vi "Conclude.vi"(8 "error in (no error)":errorcluster, 10 "Iterator Settings":T1={"Prepare timeout (ms)"=200, "Iterate timeout (ms)"=50, "Conclude timeout (ms)"=200, "Iterate period (ms)"=200, "Number of iterations"=5, "Time before stop (ms)"=5, "Active Stop Conditions"={"Number of Iterations"=FALSE, "Time Elapsed"=FALSE, "Iteration Result"=FALSE}, "Prepare Msg"=refnum, "Iterate Msg"=refnum, "Conclude Msg"=refnum, "Iterations End Report"=refnum}, 11 "Iterator Actor in":refnum<class "Iterator Actor.lvclass">) -> (0 "error out":errorcluster, 3 "Iterator Actor out":refnum<class "Iterator Actor.lvclass">)   [LabVIEW 2023, in "Iterator Actor.lvlib" / "Iterator Actor.lvclass"]
doc: "Calls the Conclude method of the Client."
uses:
  Iterator Actor.lvclass
  Abstract Iterator Actor/Iterator Settings.ctl
  Iterator Actor Abstract Messages/Iterator Report Iterations End Msg/Iterator Report Iterations End Msg.lvclass
  <vilib>/ActorFramework/Message/Message.lvclass
  Abstract Iterator Actor/Active Stop Conditions.ctl
  <vilib>/ActorFramework/Actor/Actor.lvclass/Actor.ctl
  Iterator Actor Abstract Messages/Iterator Reply Msg/Iterator Reply Msg.lvclass
  Iterator Actor Abstract Messages/Iterator Reply Msg/Iterator Reply Msg.lvclass/Iterator Reply Msg.ctl
  <vilib>/ActorFramework/Message Enqueuer/Message Enqueuer.lvclass/Message Enqueuer.ctl
  <vilib>/ActorFramework/Message Enqueuer/Enqueue.vi
  <vilib>/ActorFramework/Message Priority Queue/Priority Enqueue.vi
  Iterator Actor.lvclass/Iterator Actor.ctl
  <vilib>/ActorFramework/Actor/Actor.lvclass
  <vilib>/ErrorRing/Error Ring.xnode
  C:/Projects/Iterator Actor/Abstract Iterator Actor/Abstract Iterator Actor.lvclass
  C:/Program Files/National Instruments/LabVIEW 2023/vi.lib/LS Instruments AG/Async Methods Actor/Async Methods Actor/Async Methods Actor/Async Methods Actor.lvclass
  C:/Program Files/National Instruments/LabVIEW 2023/vi.lib/ActorFramework/Actor/Actor.lvclass
  C:/Projects/Iterator Actor/Iterator Actor/Iterator Actor/Iterator Actor.lvclass
  <vilib>/Utility/error.llb/Error Cluster From Error Code.vi
  Abstract Iterator Actor/Abstract Iterator Actor.lvclass
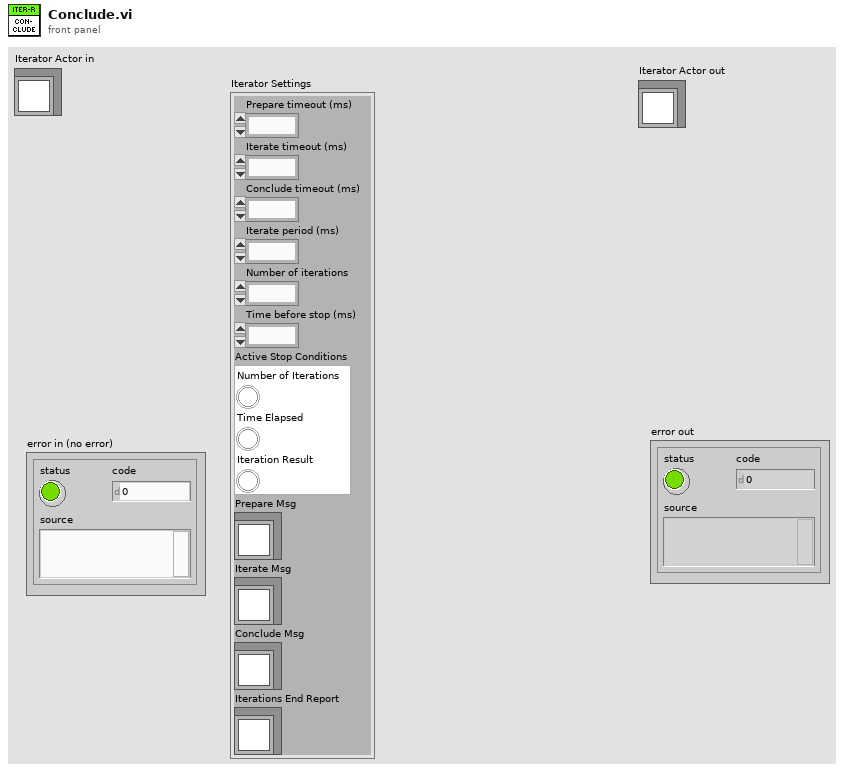
[diagram p1: front panel]
types:
  T1 = typedef "Iterator Actor.lvlib/Abstract Iterator Actor.lvclass/Iterator Settings.ctl" = cluster{"Prepare timeout (ms)":i32, "Iterate timeout (ms)":i32, "Conclude timeout (ms)":i32, "Iterate period (ms)":i32, "Number of iterations":i32, "Time before stop (ms)":i32, "Active Stop Conditions":T2, "Prepare Msg":refnum<class "Message.lvclass">, "Iterate Msg":refnum<class "Message.lvclass">, "Conclude Msg":refnum<class "Message.lvclass">, "Iterations End Report":refnum<class "Iterator Report Iterations End Msg.lvclass">}
  T2 = typedef "Iterator Actor.lvlib/Abstract Iterator Actor.lvclass/Active Stop Conditions.ctl" = cluster{"Number of Iterations":bool, "Time Elapsed":bool, "Iteration Result":bool}
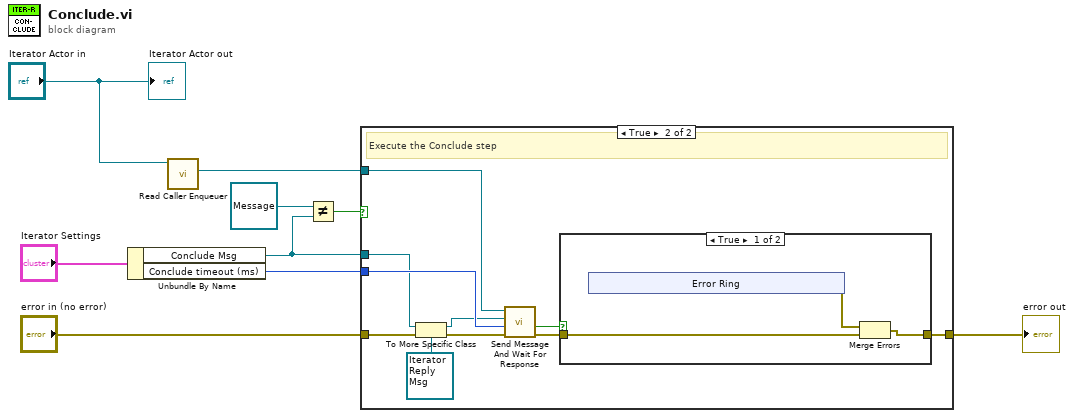
[diagram p0: block diagram]
diagram:
  n1 = Unbundle By Name("Iterator Settings") -> ("Conclude Msg"=w5:refnum<class "Message.lvclass">, "Conclude timeout (ms)"=w9:i32)
  n2 = call <vilib>:"Read Caller Enqueuer.vi"("Actor"="Iterator Actor in") -> ("Caller Enqueuer"=w3:refnum<class "Message Enqueuer.lvclass">)  [unwired: 10 in]
  n3 = Not Equal?(x=refnum<class "Message.lvclass"> refnum ("Conclude Msg"), y=w5) -> (x != y?=w4:bool)
  n4 = case shown="True" w4 {
    tunnel: w9 -> [_ w20]
    tunnel: w5 -> [_ w15]
    tunnel: w3 -> [_ w19]
    tunnel: "error in (no error)" -> [w10 w18]
    tunnel: [w10 w13] -> w6
    frame False {
      # "Caller did not configure the Conclude step.\nSkip it and go to finish."
    }
    frame True {
      # "Execute the Conclude step"
      n5 = To More Specific Class(target class=refnum<class "Iterator Reply Msg.lvclass"> refnum ("Prepare Msg"), reference=w15, error in=w18) -> (specific class reference=w14:refnum<class "Iterator Reply Msg.lvclass">, error out=w17:errorcluster)
      n6 = call "Send Message And Wait For Response.vi"("error in (no error)"=w17, "timeout in ms (-1)"=w20, "Original Message"=w14, "Message Enqueuer in"=w19) -> ("error out"=w11:errorcluster, "timed out?"=w12:bool)  [unwired: 4 in, 2 out]
      n7 = case shown="True" w12 {
        tunnel: w11 -> [w23 w28]
        tunnel: [w22 w28] -> w13
        frame True {
          n8 = xnode "Error Ring"() -> ("error out"=w21:errorcluster)
          n9 = Merge Errors(w21, w23) -> (w22:errorcluster)
        }
        frame False {
        }
      }
    }
  }
  "error out" <- w6
  "Iterator Actor out" <- "Iterator Actor in"
